vi "Weighted Variance_PN.vi"(2 "Weighted mean":dbl, 3 "weights":dbl[](array[numeric]), 4 "1D data":dbl[](array[numeric])) -> (1 "Weighted variance":dbl)   [LabVIEW 2011]
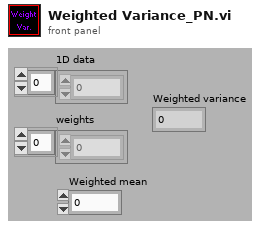
[diagram p1: front panel]
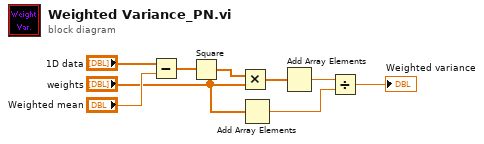
[diagram p0: block diagram]
diagram:
  n1 = Subtract(x="1D data", y="Weighted mean") -> (x-y=w7:dbl[])
  n2 = Square(x=w7) -> (x^2=w6:dbl[])
  n3 = Multiply(x=w6, y="weights") -> (x*y=w4:dbl[])
  n4 = Add Array Elements(numeric array="weights") -> (sum=w2:dbl)
  n5 = Add Array Elements(numeric array=w4) -> (sum=w3:dbl)
  n6 = Divide(x=w3, y=w2) -> (x/y=→"Weighted variance":dbl)
